vi "QuadEncCalcSGL_src.vi"(6 "dTPerSec":sgl, 8 "RevPerPulse":sgl, 10 "RevPosition":i32, 11 "AbsPosition":i32) -> (0 "RadPerSec":sgl, 1 "Theta":sgl, 2 "RevPerSec":sgl, 3 "Revolutions":sgl)   [LabVIEW 2015]
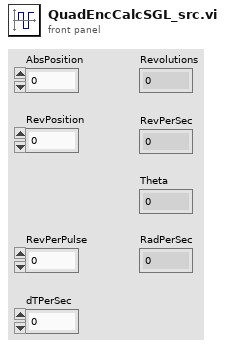
[diagram p1: front panel]
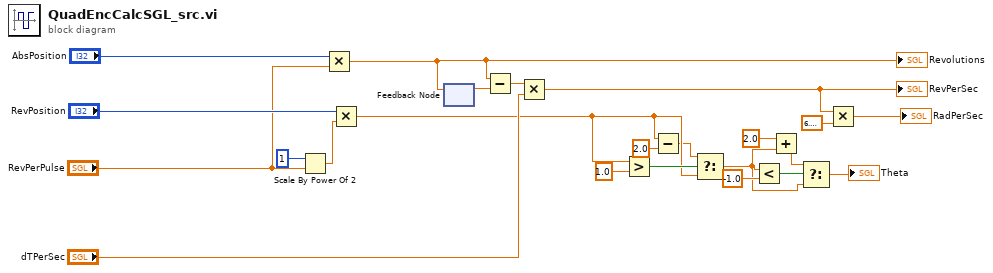
[diagram p0: block diagram]
diagram:
  n1 = Scale By Power Of 2(n=i16 1, x="RevPerPulse") -> (x*2^n=w15:sgl)
  n2 = Multiply(x="AbsPosition", y="RevPerPulse") -> (x*y=w18:sgl)
  "Revolutions" <- w18
  n3 = Multiply(x="RevPosition", y=w15) -> (x*y=w10:sgl)
  n4 = feedback-in #1(w18) -> ()
  n5 = feedback #1() -> (w21:sgl)  [unwired: 1 in]
  n6 = Subtract(x=w18, y=w21) -> (x-y=w20:sgl)
  n7 = Multiply(x=w20, y="dTPerSec") -> (x*y=w3:sgl)
  "RevPerSec" <- w3
  n8 = Greater?(x=w10, y=sgl 1.0) -> (0:w13:bool)
  n9 = Subtract(x=w10, y=sgl 2.0) -> (x-y=w8:sgl)
  n10 = Select(t=w8, s=w13, f=w10) -> (s? t:f=w6:sgl)
  n11 = Less?(x=w6, y=sgl -1.0) -> (x < y?=w11:bool)
  n12 = Add(x=sgl 2.0, y=w6) -> (x+y=w7:sgl)
  n13 = Select(t=w7, s=w11, f=w6) -> (s? t:f=→"Theta":sgl)
  n14 = Multiply(x=w3, y=sgl 6.2831855) -> (x*y=→"RadPerSec":sgl)
